vi "Image_RAW_Parse_Metadata.vi"(8 "error in (no error)":errorcluster, 11 "Metadata (U8)":u8[](array[numeric])) -> (0 "error out":errorcluster, 3 "Image Metadata":T1={"Total Block Size"=0, "Frame Index"=0, "Frame Timestamp (ns)"=0, "Lines of Pre-EBD"=0, "Lines of Image Data"=0, "Lines of Post-EBD"=0, "Bytes per Even Line"=0, "Bytes per Odd Line"=0, "Image Data Type"=44, "Frame Number"=0} {"Image Data Type" format="%x"})   [LabVIEW 2020]
uses:
  ctl/Image_Metadata.ctl
  <vilib>/Utility/error.llb/Error Cluster From Error Code.vi
  <vilib>/ErrorRing/Error Ring.xnode
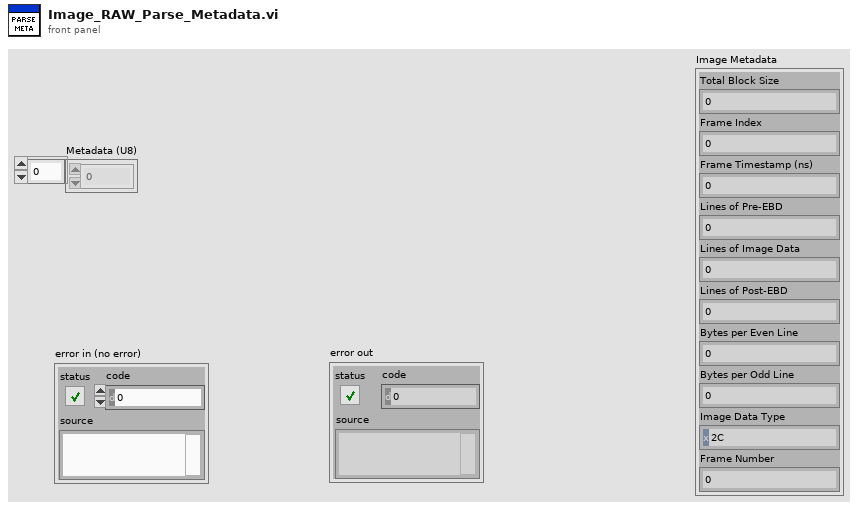
[diagram p1: front panel]
types:
  T1 = typedef "Image_Metadata.ctl" = cluster{"Total Block Size":u32, "Frame Index":u32, "Frame Timestamp (ns)":u64, "Lines of Pre-EBD":u16, "Lines of Image Data":u16, "Lines of Post-EBD":u16, "Bytes per Even Line":u16, "Bytes per Odd Line":u16, "Image Data Type":u8, "Frame Number":u16}
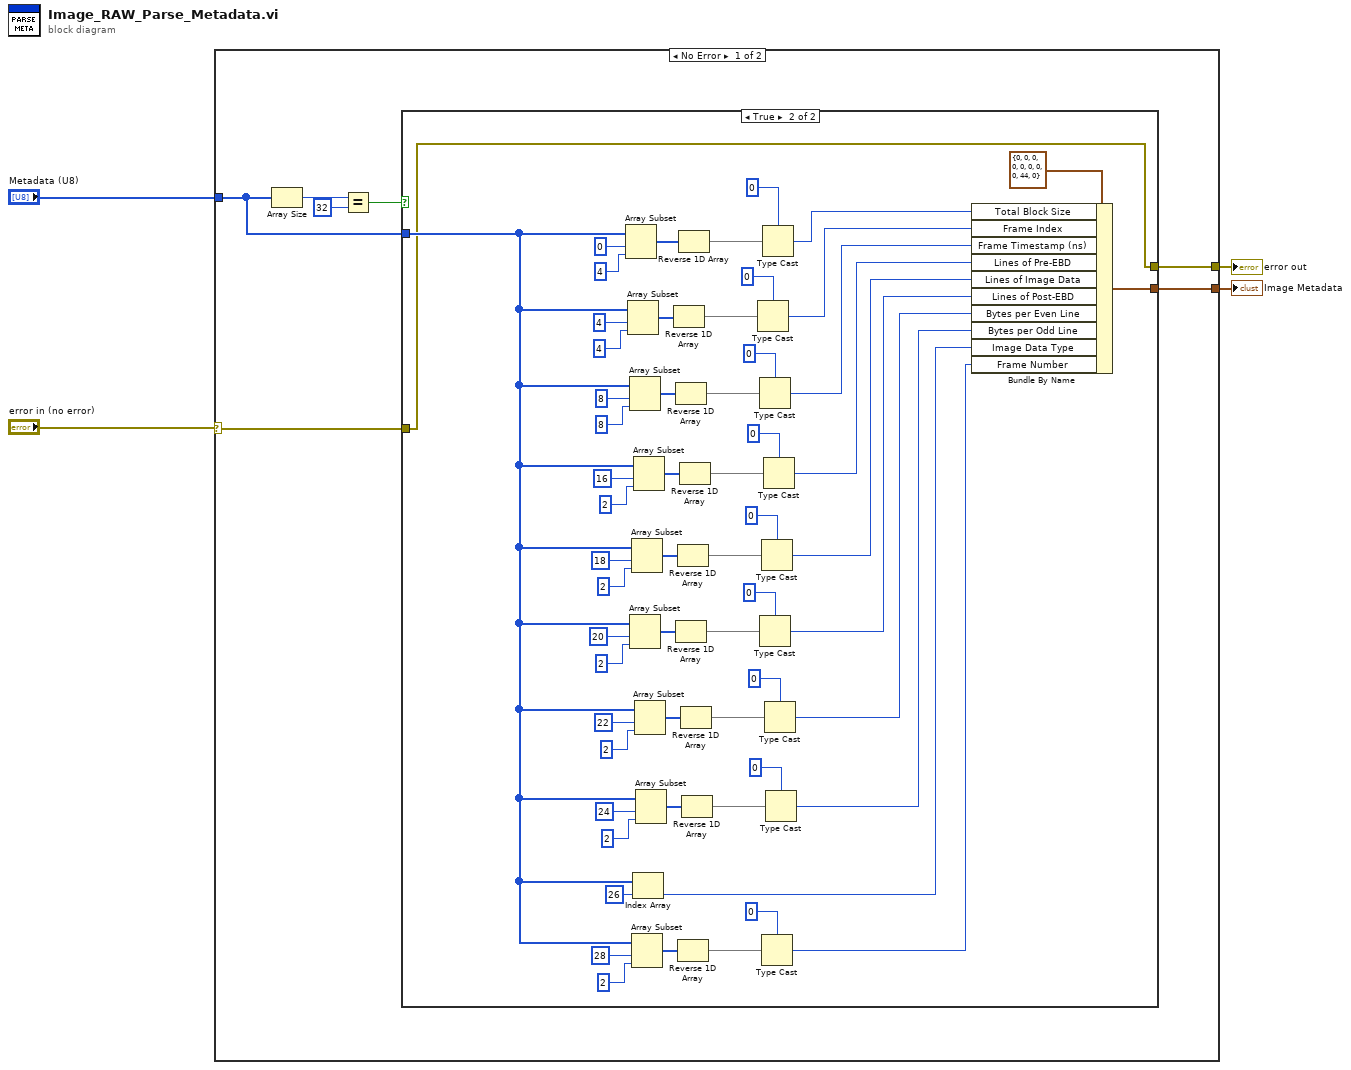
[diagram p0: block diagram]
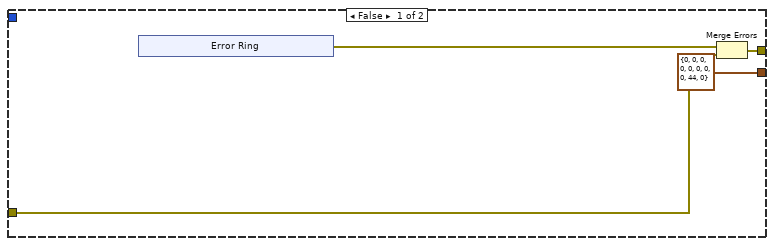
[diagram p2: hidden frame]
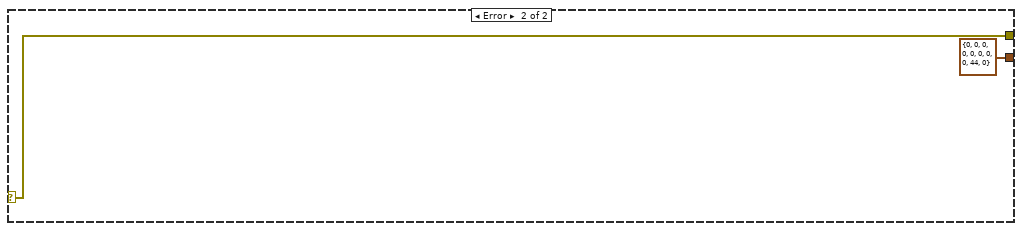
[diagram p3: hidden frame]
diagram:
  n1 = case shown="No Error" "error in (no error)" {
    selector: "error in (no error)" -> [w8 w82]
    tunnel: "Metadata (U8)" -> [w6 _]
    tunnel: [w7 w82] -> w1
    tunnel: [w5 T1 {"Total Block Size"=0, "Frame Index"=0, "Frame Timestamp (ns)"=0, "Lines of Pre-EBD"=0, "Lines of Image Data"=0, "Lines of Post-EBD"=0, "Bytes per Even Line"=0, "Bytes per Odd Line"=0, "Image Data Type"=44, "Frame Number"=0} ("Image Metadata")] -> w2
    frame No Error {
      n2 = Array Size(array=w6) -> (size(s)=w11:i32)
      n3 = Equal?(x=w11, y=32) -> (x = y?=w9:bool)
      n4 = case shown="True" w9 {
        tunnel: w8 -> [w14 w21]
        tunnel: [w13 w21] -> w7
        tunnel: w6 -> [_ w25]
        tunnel: [T1 {"Total Block Size"=0, "Frame Index"=0, "Frame Timestamp (ns)"=0, "Lines of Pre-EBD"=0, "Lines of Image Data"=0, "Lines of Post-EBD"=0, "Bytes per Even Line"=0, "Bytes per Odd Line"=0, "Image Data Type"=44, "Frame Number"=0} ("Image Metadata") w22] -> w5
        frame False {
          n5 = xnode "Error Ring"() -> ("error out"=w15:errorcluster)
          n6 = Merge Errors(w15, w14) -> (w13:errorcluster)
        }
        frame True {
          n7 = Array Subset(array=w25, index=0, length=4) -> (w78:u8[])
          n8 = Array Subset(array=w25, index=4, length=4) -> (w69:u8[])
          n9 = Array Subset(array=w25, index=8, length=8) -> (w63:u8[])
          n10 = Array Subset(array=w25, index=20, length=2) -> (w46:u8[])
          n11 = Array Subset(array=w25, index=18, length=2) -> (w52:u8[])
          n12 = Array Subset(array=w25, index=28, length=2) -> (w26:u8[])
          n13 = Index Array(array=w25, index=26) -> (element=w30:u8)
          n14 = Array Subset(array=w25, index=16, length=2) -> (w58:u8[])
          n15 = Array Subset(array=w25, index=22, length=2) -> (w40:u8[])
          n16 = Array Subset(array=w25, index=24, length=2) -> (w34:u8[])
          n17 = Reverse 1D Array(array=w69) -> (reversed array=w70:u8[])
          n18 = Reverse 1D Array(array=w63) -> (reversed array=w64:u8[])
          n19 = Reverse 1D Array(array=w46) -> (reversed array=w47:u8[])
          n20 = Reverse 1D Array(array=w52) -> (reversed array=w53:u8[])
          n21 = Reverse 1D Array(array=w26) -> (reversed array=w27:u8[])
          n22 = Reverse 1D Array(array=w78) -> (reversed array=w76:u8[])
          n23 = Reverse 1D Array(array=w58) -> (reversed array=w59:u8[])
          n24 = Reverse 1D Array(array=w40) -> (reversed array=w41:u8[])
          n25 = Reverse 1D Array(array=w34) -> (reversed array=w35:u8[])
          n26 = Type Cast(type=u32 0, x=w70) -> (*(type *) &x=w68:u32)
          n27 = Type Cast(type=u64 0, x=w64) -> (*(type *) &x=w62:u64)
          n28 = Type Cast(type=u16 0, x=w47) -> (*(type *) &x=w44:u16)
          n29 = Type Cast(type=u16 0, x=w53) -> (*(type *) &x=w50:u16)
          n30 = Type Cast(type=u16 0, x=w27) -> (*(type *) &x=w23:u16)
          n31 = Type Cast(type=u32 0, x=w76) -> (*(type *) &x=w74:u32)
          n32 = Type Cast(type=u16 0, x=w59) -> (*(type *) &x=w56:u16)
          n33 = Type Cast(type=u16 0, x=w41) -> (*(type *) &x=w38:u16)
          n34 = Type Cast(type=u16 0, x=w35) -> (*(type *) &x=w32:u16)
          n35 = Bundle By Name(cluster=T1 {"Total Block Size"=0, "Frame Index"=0, "Frame Timestamp (ns)"=0, "Lines of Pre-EBD"=0, "Lines of Image Data"=0, "Lines of Post-EBD"=0, "Bytes per Even Line"=0, "Bytes per Odd Line"=0, "Image Data Type"=44, "Frame Number"=0} ("Image Metadata"), "Total Block Size"=w74, "Frame Index"=w68, "Frame Timestamp (ns)"=w62, "Lines of Pre-EBD"=w56, "Lines of Image Data"=w50, "Lines of Post-EBD"=w44, "Bytes per Even Line"=w38, "Bytes per Odd Line"=w32, "Image Data Type"=w30, "Frame Number"=w23) -> (w22:T1)
        }
      }
    }
    frame Error {
    }
  }
  "error out" <- w1
  "Image Metadata" <- w2
